vi "加载所有企业与用户信息.vi"(11 "个人剂量仪-云服务器.i":refnum<class "个人剂量仪-云服务器.lvclass">) -> (1 "获取成功？":bool, 3 "个人剂量仪-云服务器.o":refnum<class "个人剂量仪-云服务器.lvclass">)   [LabVIEW 2013, in "个人剂量仪-云服务器.lvclass"]
uses:
  <vilib>/addons/database/Connection.llb/Conn Execute.vi
  <vilib>/addons/database/NI_Database_API.lvlib
panel:
  out "列名（参考）":T1(ring)
  out "所有企业名":string[](array[string])
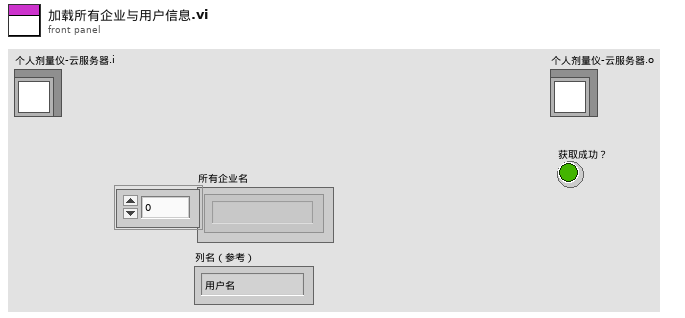
[diagram p1: front panel]
types:
  T1 = enum16{"用户名", "设备MAC", "设备状态", "密码", "职类", "姓名", "电话", "邮箱", "备注", "最后活动"}
  T2 = typedef "NI_Database_API.lvlib/Conn ObjectReference.ctl" = refnum<k1>
  T3 = cluster{"企业信息":cluster{"登录名":string, "密码":string, "企业名称":string, "邮箱":string, "电话":string}, "用户列表":cluster{"用户名":string, "设备MAC":string, "设备状态":dbl, "密码":string, "职类":dbl, "姓名":string, "电话":string, "邮箱":string, "备注":string, "最后活动":string}[]}
  T4 = cluster{"用户名":string, "设备MAC":string, "设备状态":i32, "密码":string, "职类":i32, "姓名":string, "电话":string, "邮箱":string, "备注":string, "最后活动":string}
  T5 = cluster{"登录名":string, "密码":string, "企业名称":string, "邮箱":string, "电话":string}
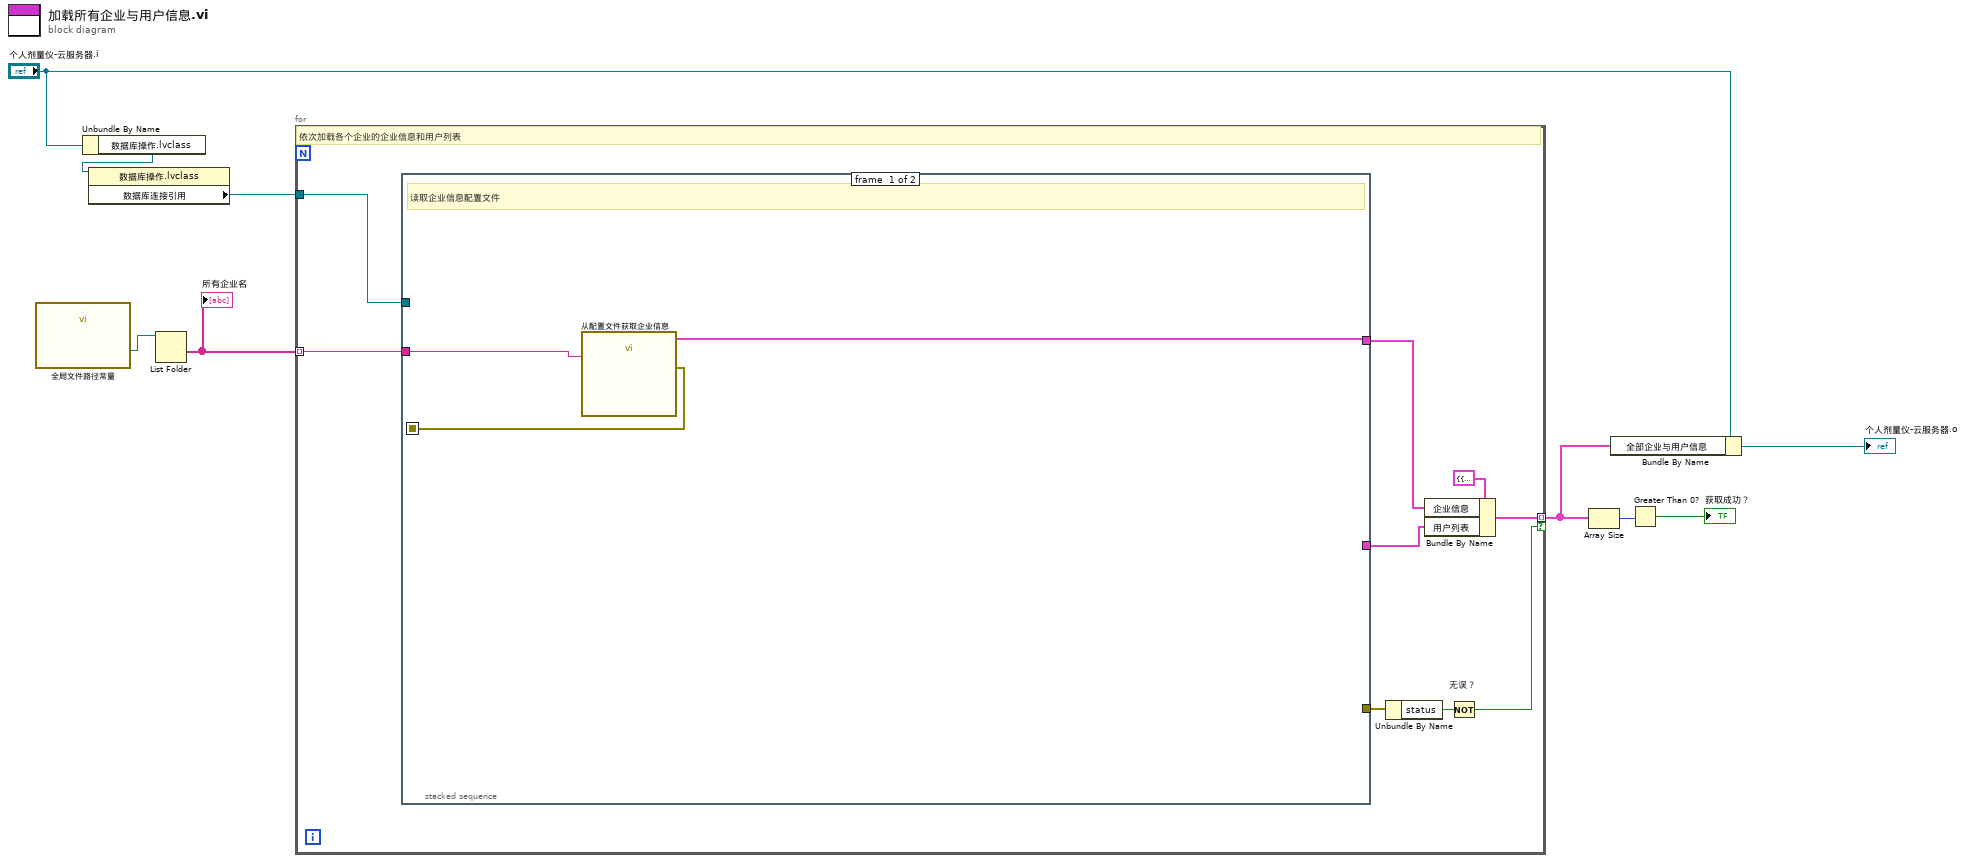
[diagram p0: block diagram]
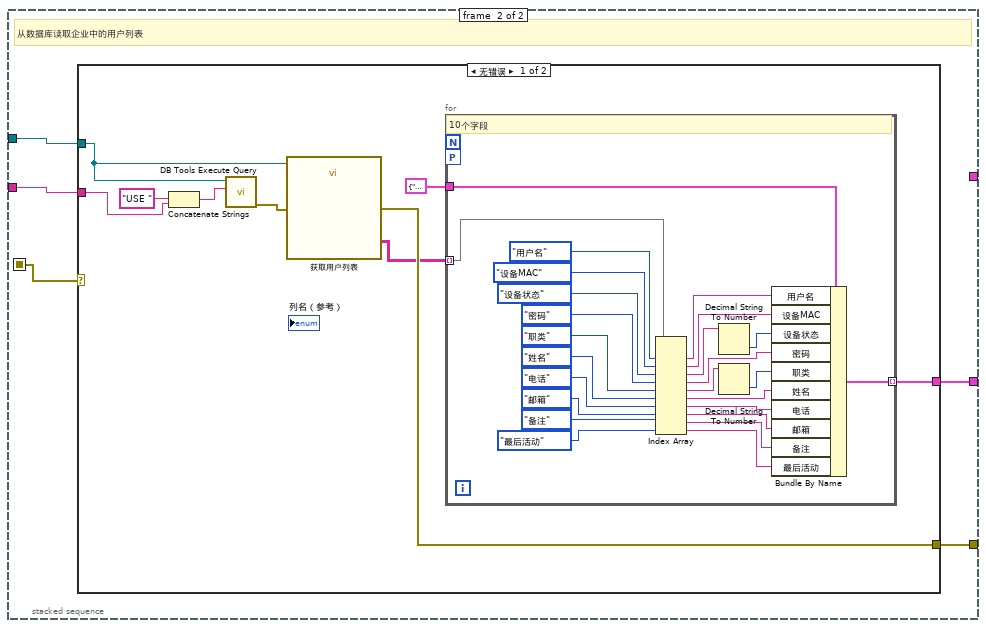
[diagram p2: hidden frame]
diagram:
  n1 = call "全局文件路径常量.vi"() -> ("用户数据库根目录"=w9:path)  [unwired: 9 in, 2 out]
  n2 = Unbundle By Name("个人剂量仪-云服务器.i") -> ("数据库操作.lvclass"=w6:refnum<class "数据库操作.lvclass">)
  n3 = property class="数据库操作.lvclass"(reference=w6) -> ("数据库连接引用"=w5:T2)  [unwired: 1 in, 2 out]
  n4 = List Folder(path=w9) -> (folder names=w8:string[])  [unwired: 3 in, 3 out]
  "所有企业名" <- w8
  n5 = for {
    tunnel: w8 -> [w18] mode=indexing
    tunnel: w5 -> [w17]
    tunnel: [w11] -> w3 mode=indexing if=w10
    # "依次加载各个企业的企业信息和用户列表"
    n6 = stacked-sequence {
      seq-local: [w19 _] -> [_ w24]
      tunnel: w18 -> [w21 w26]
      tunnel: [w20 _] -> w15
      tunnel: w17 -> [_ w25]
      tunnel: [_ w23] -> w14
      tunnel: [_ w22] -> w12
      frame #0 {
        # "读取企业信息配置文件"
        n7 = call "从配置文件获取企业信息.vi"("登录名"=w21) -> ("error out"=w19:errorcluster, "企业信息"=w20:T5)  [unwired: 9 in]
      }
      frame #1 {
        # "从数据库读取企业中的用户列表"
        n8 = case shown="无错误" w24 {
          selector: w24 -> [_ w61]
          tunnel: w26 -> [w33 _]
          tunnel: w25 -> [w32 _]
          tunnel: [w30 w61] -> w23
          tunnel: [w27 _] -> w22
          frame No Error {
            n9 = Concatenate Strings("USE ", w33) -> (w35:string)
            n10 = call-poly <vilib>:"DB Tools Execute Query.vi"("SQL query"=w35, "connection reference"=w32) -> ("error out"=w31:errorcluster)  [unwired: 6 in, 1 out]
            n11 = call "获取用户列表.vi"("error in (no error)"=w31, "数据库连接引用"=w32) -> ("用户列表"=w29:string[][], "error out"=w30:errorcluster)  [unwired: 4 in, 4 out]
            n12 = for {
              tunnel: w29 -> [w60] mode=indexing
              tunnel: T4 {"用户名"="", "设备MAC"="", "设备状态"=0, "密码"="", "职类"=0, "姓名"="", "电话"="", "邮箱"="", "备注"="", "最后活动"=""} ("设备绑定信息") -> [w49]
              workers-P: _ -> [_]
              tunnel: [w36] -> w27 mode=indexing
              # "10个字段"
              n13 = Index Array(array=w60, index #1=T1."用户名", index #2=T1."设备MAC", index #3=T1."设备状态", index #4=T1."密码", index #5=T1."职类", index #6=T1."姓名", index #7=T1."电话", index #8=T1."邮箱", index #9=T1."备注", index #10=T1."最后活动") -> (element #1=w48:string, element #2=w47:string, element #3=w40:string, element #4=w46:string, element #5=w38:string, element #6=w45:string, element #7=w44:string, element #8=w43:string, element #9=w42:string, element #10=w41:string)
              n14 = Decimal String To Number(string=w40) -> (number=w39:i32)  [unwired: 2 in, 1 out]
              n15 = Decimal String To Number(string=w38) -> (number=w37:i32)  [unwired: 2 in, 1 out]
              n16 = Bundle By Name(cluster=w49, "用户名"=w48, "设备MAC"=w47, "设备状态"=w39, "密码"=w46, "职类"=w37, "姓名"=w45, "电话"=w44, "邮箱"=w43, "备注"=w42, "最后活动"=w41) -> (w36:T4)
            }
          }
          frame Error {
          }
        }
      }
    }
    n17 = Unbundle By Name(w14) -> ("status"=w13:bool)
    n18 = Bundle By Name(cluster=T3 {"企业信息"={"登录名"="", "密码"="", "企业名称"="", "邮箱"="", "电话"=""}, "用户列表"=[]} ("企业与用户信息"), "企业信息"=w15, "用户列表"=w12) -> (w11:T3)
    n19 = Not "无误？"(x=w13) -> (.not. x?=w10:bool)
  }
  n20 = Array Size(array=w3) -> (size(s)=w2:i32)
  n21 = Bundle By Name(cluster="个人剂量仪-云服务器.i", "全部企业与用户信息"=w3) -> (→"个人剂量仪-云服务器.o":refnum<class "个人剂量仪-云服务器.lvclass">)
  n22 = Greater Than 0?(x=w2) -> (x > 0?=→"获取成功？":bool)
